vi "Update Sample History.vi"(10 "R in":T1, 11 "Sample":T1) -> (2 "covariance matrix V":T1, 3 "R out":T1, 5 "Sample Unwrapped":T1)   [LabVIEW 2017]
uses:
  <vilib>/gmath/NI_Gmath.lvlib
  <vilib>/Analysis/Matrix/Datatypes/RealMatrix.ctl
  <vilib>/Analysis/Matrix/NI_Matrix.lvlib
  <vilib>/Analysis/NI_AALPro.lvlib
  <vilib>/Analysis/Matrix/Numeric/Multiply/Multiply - RM,R.vi
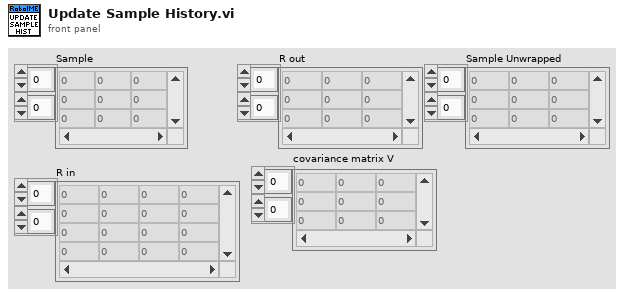
[diagram p1: front panel]
types:
  T1 = typedef "NI_Matrix.lvlib/RealMatrix.ctl" = dbl[][]
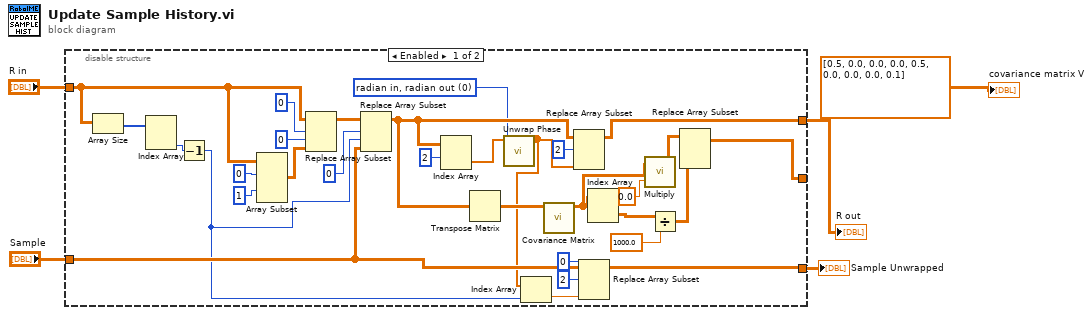
[diagram p0: block diagram]
diagram:
  n1 = disable-structure shown="Enabled" {
    disable-tunnel: "Sample" -> [w17 _]
    disable-tunnel: "R in" -> [w20 w37]
    disable-tunnel: [w22 w37] -> w3
    disable-tunnel: [w11 _] -> w2
    disable-tunnel: [w6 _] -> _
    frame Enabled {
      w21 = 0 items=["radian in, radian out", "radian in, degree out", "degree in, degree out", "degree in, radian out"] ("phase unit")
      n2 = Array Size(array=w20) -> (size(s)=w19:i32[])
      n3 = Index Array(array=w19) -> (element #2=w18:i32)  [unwired: 2 in, 1 out]
      n4 = Decrement(x=w18) -> (x-1=w15:i32)
      n5 = Array Subset(array=w20, index (row)=0 ("index"), index (col)=1 ("index")) -> (w33:T1)  [unwired: 2 in]
      n6 = Replace Array Subset(array=w20, new element=w33, index (row)=0 ("disabled index (row)"), index (col)=0 ("disabled index (col)")) -> (w36:T1)
      n7 = Replace Array Subset(array=w36, new element=w17, index (row)=0, index (col)=w15) -> (w24:T1)
      n8 = Index Array(array=w24, index (row)=2) -> (element=w25:dbl[])  [unwired: 1 in]
      n9 = Transpose Matrix(1:w24) -> (0:w29:T1)
      n10 = call <vilib>:"Unwrap Phase.vi"("phase unit"=w21, "Phase"=w25) -> ("Unwrapped Phase"=w16:dbl[])  [unwired: 8 in, 1 out]
      n11 = Index Array(array=w16, index=w15) -> (element=w13:dbl)
      n12 = call <vilib>:"Covariance Matrix.vi"("X"=w29) -> ("covariance matrix V"=w10:T1)  [unwired: 9 in, 1 out]
      n13 = Replace Array Subset(array=w24, new element=w16, index (row)=2) -> (w22:T1)  [unwired: 1 in]
      n14 = Replace Array Subset(array=w17, new element=w13, index (row)=2, index (col)=0 ("disabled index (col)")) -> (w11:T1)
      n15 = Index Array(array=w10) -> (element=w27:T1)  [unwired: 2 in]
      n16 = call-poly <vilib>:"Multiply.vi"("Real Scalar c"=0.0 ("Real Matrix B"), "Real Matrix A"=w10) -> ("A * c"=w8:T1)
      n17 = Divide(x=w27, y=1000.0) -> (x/y=w7:T1)
      n18 = Replace Array Subset(array=w8, new element=w7) -> (w6:T1)  [unwired: 2 in]
    }
    frame Disabled {
    }
  }
  "R out" <- w3
  "Sample Unwrapped" <- w2
  "covariance matrix V" <- T1 [[0.5, 0.0, 0.0], [0.0, 0.5, 0.0], [0.0, 0.0, 0.1]] ("matrix")
